vi "Convert Pot Volts to Degrees.vi"() -> ()   [LabVIEW 2014, in "hhVI.lvlib"]
uses:
  hhVI.lvlib
panel:
  out "degrees":dbl
  in  "voltage":dbl
  in  "Max rotation (degrees)":dbl
  in  "Min (volts)":dbl
  in  "Max (volts)":dbl
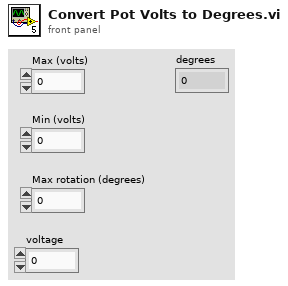
[diagram p1: front panel]
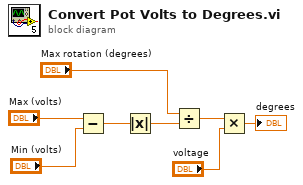
[diagram p0: block diagram]
diagram:
  n1 = Subtract(x="Max (volts)", y="Min (volts)") -> (x-y=w6:dbl)
  n2 = Absolute Value(x=w6) -> (abs(x)=w2:dbl)
  n3 = Divide(x="Max rotation (degrees)", y=w2) -> (x/y=w5:dbl)
  n4 = Multiply(x=w5, y="voltage") -> (x*y=→"degrees":dbl)
